vi "Duplicate.vi"(8 "error in":errorcluster, 10 "parameters":variant, 11 "node in":refnum<class "TBM Configuration Node.lvclass">) -> (0 "error out":errorcluster, 3 "node copy out":refnum<class "TBM Configuration Node.lvclass">)   [LabVIEW 2013, in "PL Framework Configuration Tool.lvlib" / "TBM Configuration Node.lvclass"]
doc: "Implements the specific behavior of a node when it is being duplicated\nCan be used to change the name of the new node for example adding Copy to it."
uses:
  TBM Configuration Node.lvclass
  <vilib>/NI/Tag Bus Module Framework/root configuration/TBM configuration.lvclass
  <vilib>/NI/CEF/CEF_TreeControl/serializable configuration/NISE_CEF_serializable configuration.lvclass
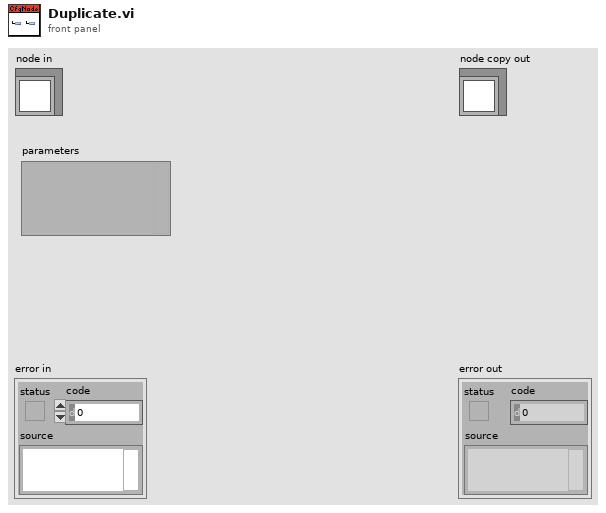
[diagram p1: front panel]
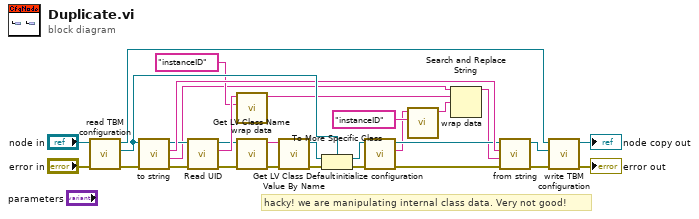
[diagram p0: block diagram]
diagram:
  # "hacky! we are manipulating internal class data. Very not good!"
  n1 = call-dynamic "read TBM configuration.vi"("error in"="error in", "TBM Configuration Node in"="node in") -> ("error out"=w28:errorcluster, "configuration"=w24:refnum<class "TBM configuration.lvclass">, "TBM Configuration Node out"=w20:refnum<class "TBM Configuration Node.lvclass">)  [unwired: 7 in]
  n2 = call-dynamic "to string.vi"("error in"=w28, "configuration in"=w24) -> ("error out"=w11:errorcluster, "data"=w4:string, "version"=w15:string, "configuration out"=w10:refnum<class "TBM configuration.lvclass">)  [unwired: 6 in]
  n3 = call <vilib>:"Read UID.vi"("error in"=w11, "configuration in"=w10) -> ("error out"=w8:errorcluster, "instance id"=w14:string, "configuration out"=w9:refnum<class "TBM configuration.lvclass">)  [unwired: 7 in]
  n4 = call <vilib>:"wrap data.vi"("identifier"="instanceID" ("additional identifier"), "data to wrap"=w14) -> ("wrapped data"=w2:string)  [unwired: 9 in]
  n5 = call <vilib>:"Get LV Class Name.vi"("error in (no error)"=w8, "object"=w9) -> ("error out"=w26:errorcluster, "class name"=w27:string)  [unwired: 8 in]
  n6 = call <vilib>:"Get LV Class Default Value By Name.vi"("error in (no error)"=w26, "class name"=w27) -> ("error out"=w25:errorcluster, "object"=w23:refnum<class>)  [unwired: 8 in]
  n7 = To More Specific Class(target class=w24, reference=w23, error in=w25) -> (specific class reference=w21:refnum<class "TBM configuration.lvclass">, error out=w22:errorcluster)
  n8 = call-dynamic "initialize configuration.vi"("error in"=w22, "configuration in"=w21) -> ("error out"=w6:errorcluster, "instance identifier"=w5:string, "configuration out"=w7:refnum<class "TBM configuration.lvclass">)  [unwired: 7 in]
  n9 = call <vilib>:"wrap data.vi"("identifier"="instanceID" ("additional identifier"), "data to wrap"=w5) -> ("wrapped data"=w1:string)  [unwired: 9 in]
  n10 = Search and Replace String(input string=w4, search string=w2, replace string=w1) -> (result string=w3:string)  [unwired: 5 in, 3 out]
  n11 = call-dynamic "from string.vi"("error in"=w6, "data"=w3, "version"=w15, "configuration in"=w7) -> ("error out"=w19:errorcluster, "configuration out"=w16:refnum<class "TBM configuration.lvclass">)  [unwired: 6 in]
  n12 = call-dynamic "write TBM configuration.vi"("error in"=w19, "configuration"=w16, "TBM Configuration Node in"=w20) -> ("error out"=→"error out":errorcluster, "TBM Configuration Node out"=→"node copy out":refnum<class "TBM Configuration Node.lvclass">)  [unwired: 7 in]
